vi "EMV High T7 Temperature Check.vi"(8 "error in (no error)":errorcluster, 10 "Abnormal Input Temperature":dbl=90.0, 11 "T7 History":dbl[](array[numeric])) -> (0 "error out":errorcluster, 2 "Hot Inlet Water?":bool, 3 "T6 History Output":dbl[](array[numeric]))   [LabVIEW 2020]
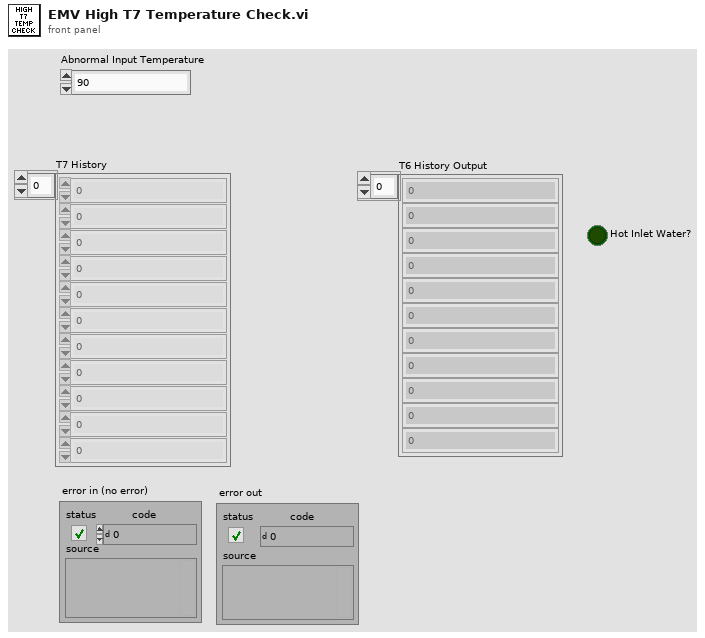
[diagram p1: front panel]
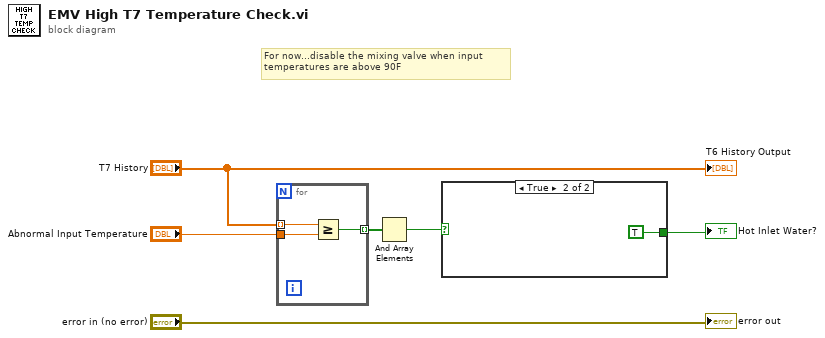
[diagram p0: block diagram]
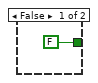
[diagram p2: hidden frame]
diagram:
  # "For now...disable the mixing valve when input \ntemperatures are above 90F"
  n1 = for {
    tunnel: "T7 History" -> [w9] mode=indexing
    tunnel: "Abnormal Input Temperature" -> [w8]
    tunnel: [w7] -> w3 mode=indexing
    n2 = Greater Or Equal?(x=w9, y=w8) -> (x >= y?=w7:bool)
  }
  n3 = And Array Elements(Boolean array=w3) -> (logical AND=w2:bool)
  n4 = case shown="True" w2 {
    tunnel: [FALSE TRUE] -> w6
    frame False {
    }
    frame True {
    }
  }
  "Hot Inlet Water?" <- w6
  "error out" <- "error in (no error)"
  "T6 History Output" <- "T7 History"
